vi "传感器读取.vi"() -> ()   [LabVIEW 2020]
uses:
  <vilib>/Instr/_visa.llb/VISA Configure Serial Port (Instr).vi
  Global_Variable/Global.vi
  Global_Variable/A131258.vi
panel:
  out "error out":cluster{"status":bool, "code":i32} caption="错误输出"
  in  "error in (no error)":errorcluster caption="错误输入（无错误）"
  out "数值 4":dbl format="%#_13g"
  out "数值 2":dbl format="%#_13g"
  in  "停止":bool
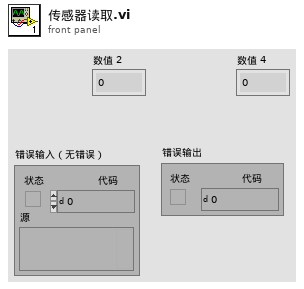
[diagram p1: front panel]
types:
  T1 = cluster{"左平均扭矩":cluster{"正转":dbl, "反转":dbl}, "左矩波动":cluster{"正转":dbl, "反转":dbl}, "左空载":cluster{"正转":dbl, "反转":dbl}, "右平均扭矩":cluster{"正转":dbl, "反转":dbl}, "右扭矩波动":cluster{"正转":dbl, "反转":dbl}, "右空载":cluster{"正转":dbl, "反转":dbl}, "扭矩对称":cluster{"左":dbl, "右":dbl}, "左零点漂移":cluster{"正":dbl, "反":dbl}, "右零点漂移":cluster{"正":dbl, "反":dbl}}
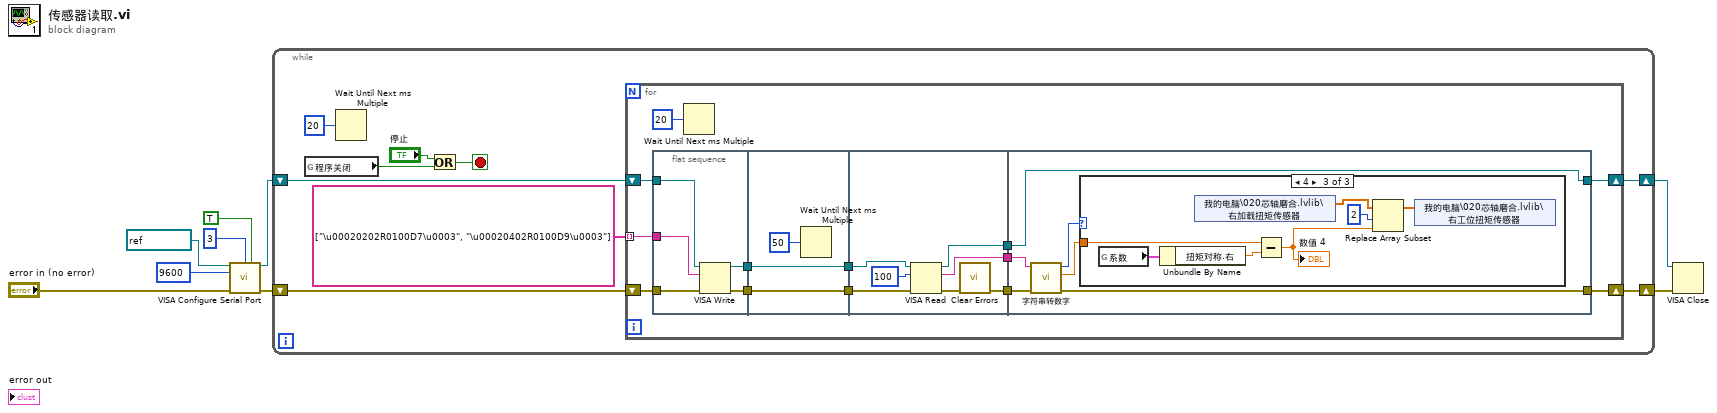
[diagram p0: block diagram]
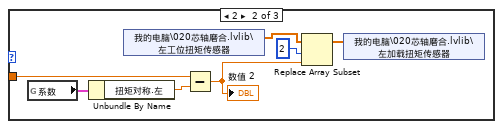
[diagram p3: hidden frame]
diagram:
  n1 = call-poly "VISA Configure Serial Port"("VISA resource name"=refnum<visa-resource-name> "COM8", "termination char\n(0xA = '\\n' = LF)"=u8 3 ("termination char\n(0xA = '\\n' = LF)"), "Enable Termination\nChar (T)"=TRUE ("Enable Termination\nChar (T)"), "baud rate (9600)"=u32 9600, "error in (no error)"="error in (no error)") -> ("VISA resource name out"=w4:refnum<visa-resource-name>, "error out"=w2:errorcluster)  [unwired: 9 in]
  n2 = while {
    shift-right: [w16] -> w9
    shift-left: w4 -> [w17]
    shift-right: [w13] -> w7
    shift-left: w2 -> [w14]
    stop <- w11 stop-if-true
    n3 = global read "Global.vi" "程序关闭"() -> (w10:bool)
    n4 = Wait Until Next ms Multiple(millisecond multiple=u32 20 ("毫秒倍数")) -> ()  [unwired: 1 out]
    n5 = Or(x="停止", y=w10) -> (x .or. y?=w11:bool)
    n6 = for {
      tunnel: string[] ["\u00020202R0100D7\u0003", "\u00020402R0100D9\u0003"] ("写入缓冲区") -> [w30] mode=indexing
      shift-right: [w21] -> w16
      shift-left: w17 -> [w31]
      shift-right: [w19] -> w13
      shift-left: w14 -> [w29]
      n7 = flat-sequence {
        tunnel: w31 -> [w36]
        tunnel: w30 -> [w34]
        tunnel: w29 -> [w33]
        tunnel: [w35] -> w28
        tunnel: [w32] -> w27
        tunnel: w28 -> [w39]
        tunnel: w27 -> [w38]
        tunnel: [w39] -> w26
        tunnel: [w38] -> w25
        tunnel: w26 -> [w44]
        tunnel: w25 -> [w46]
        tunnel: [w40] -> w24
        tunnel: [w42] -> w23
        tunnel: [w41] -> w22
        tunnel: [w52] -> w21
        tunnel: [w49] -> w19
        tunnel: w24 -> [w50]
        tunnel: w23 -> [w51]
        tunnel: w22 -> [w52]
        frame #0 {
          n8 = VISA Write(VISA resource name=w36, write buffer=w34, error in (no error)=w33) -> (VISA resource name out=w35:refnum<visa-resource-name>, error out=w32:errorcluster)  [unwired: 1 out]
        }
        frame #1 {
          n9 = Wait Until Next ms Multiple(millisecond multiple=u32 50 ("毫秒倍数")) -> ()  [unwired: 1 out]
        }
        frame #2 {
          n10 = VISA Read(VISA resource name=w44, byte count=u32 100 ("字节总数"), error in (no error)=w46) -> (VISA resource name out=w41:refnum<visa-resource-name>, read buffer=w42:string, error out=w43:errorcluster)  [unwired: 1 out]
          n11 = call <vilib>:"Clear Errors.vi"("error in (no error)"=w43) -> ("error out"=w40:errorcluster)  [unwired: 5 in, 1 out]
        }
        frame #3 {
          n12 = call "字符串转数字.vi"("error in (no error)"=w50, "字符串"=w51) -> ("error out"=w49:errorcluster, "数值"=w47:dbl, "ID"=w48:i32)  [unwired: 7 in]
          n13 = case shown="4" w48 {
            tunnel: w47 -> [_ w56 w64]
            frame 0, Default {
            }
            frame 2 {
              n14 = global read "A131258.vi" "系数"() -> (w55:T1)
              n15 = Unbundle By Name(w55) -> ("扭矩对称.左"=w53:dbl)
              n16 = shared-variable "我的电脑\\020芯轴磨合.lvlib\\左工位扭矩传感器"() -> (w57:sgl[])  [unwired: 1 in, 1 out]
              n17 = Subtract(x=w56, y=w53) -> (x-y=w54:dbl)
              "数值 2" <- w54
              n18 = Replace Array Subset(array=w57, new element=w54, index=2 ("索引")) -> (w58:sgl[])
              n19 = shared-variable "我的电脑\\020芯轴磨合.lvlib\\左加载扭矩传感器"(w58) -> ()  [unwired: 1 in, 1 out]
            }
            frame 4 {
              n20 = global read "A131258.vi" "系数"() -> (w63:T1)
              n21 = Unbundle By Name(w63) -> ("扭矩对称.右"=w61:dbl)
              n22 = shared-variable "我的电脑\\020芯轴磨合.lvlib\\右加载扭矩传感器"() -> (w66:sgl[])  [unwired: 1 in, 1 out]
              n23 = Subtract(x=w64, y=w61) -> (x-y=w62:dbl)
              "数值 4" <- w62
              n24 = Replace Array Subset(array=w66, new element=w62, index=2 ("索引")) -> (w60:sgl[])
              n25 = shared-variable "我的电脑\\020芯轴磨合.lvlib\\右工位扭矩传感器"(w60) -> ()  [unwired: 1 in, 1 out]
            }
          }
        }
      }
      n26 = Wait Until Next ms Multiple(millisecond multiple=u32 20 ("毫秒倍数")) -> ()  [unwired: 1 out]
    }
  }
  n27 = VISA Close(VISA resource name=w9, error in (no error)=w7) -> ()  [unwired: 1 out]
